vi "Tic-Tac-Toe-PerfectAI.vi"() -> ()   [LabVIEW 2013]
uses:
  Typedef/Board.ctl
  Typedef/Cell.ctl
  Typedef/AI Table Node.ctl
panel:
  in  "Blue AI":bool
  in  "Red AI":bool
  out "Blue":bool
  out "Red":bool
  out "Board":T1={"0,0"=enum."X", "1,0"=enum."X", "2,0"=enum."X", "0,1"=enum."X", "1,1"=enum."X", "2,1"=enum."X", "0,2"=enum."X", "1,2"=enum."", "2,2"=enum."X"}
  # "Turn"
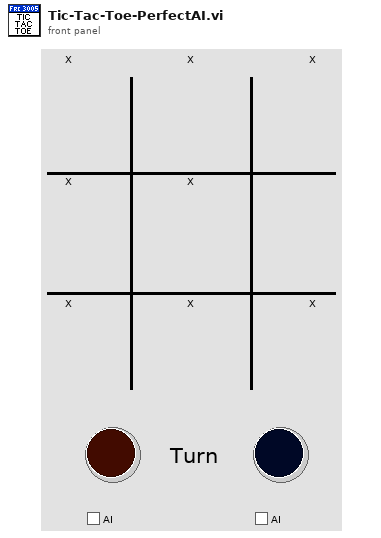
[diagram p1: front panel]
types:
  T1 = typedef "Board.ctl" = cluster{"0,0":T2, "1,0":T2, "2,0":T2, "0,1":T2, "1,1":T2, "2,1":T2, "0,2":T2, "1,2":T2, "2,2":T2}
  T2 = typedef "Cell.ctl" = enum16{"", "X", "O"}
  T3 = cluster{"Selected Row":i32, "Selected Column":i32, "Team":bool, "AI Table Head":i32, "AI Table Const":i32}
  T4 = typedef "AI Table Node.ctl" = cluster{"Board State":i32, "Child Nodes":i32[], "X PCT":dbl, "O PCT":dbl, "Index":i32}
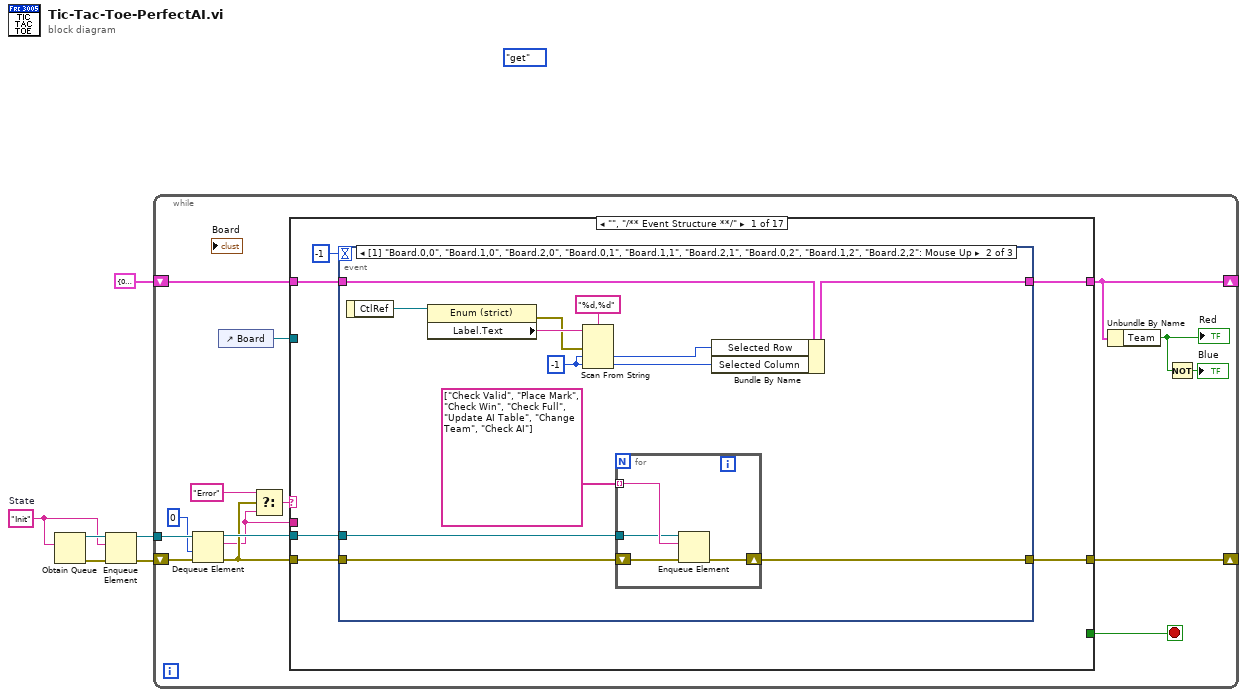
[diagram p0: block diagram]
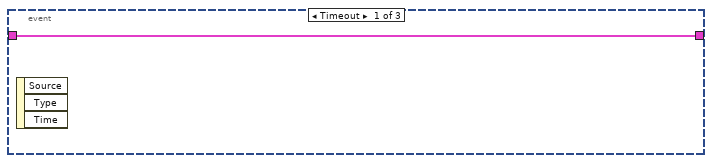
[diagram p2: hidden frame]
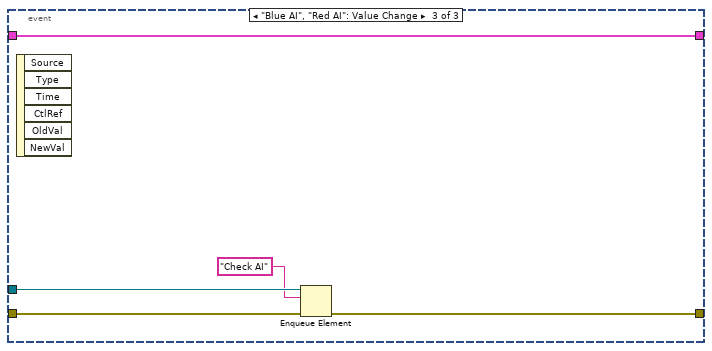
[diagram p3: hidden frame]
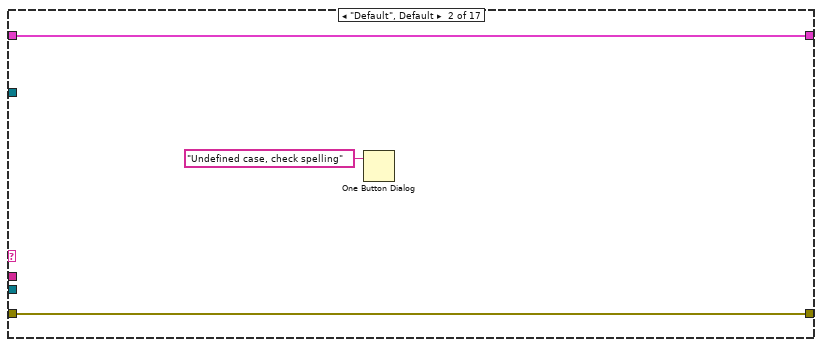
[diagram p4: hidden frame]
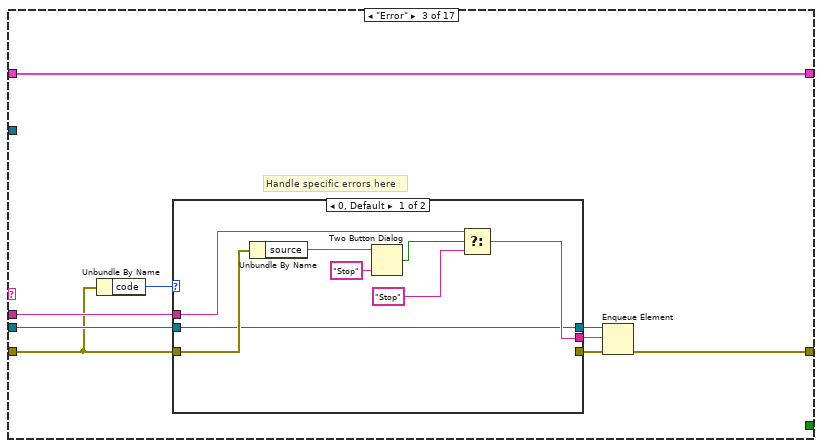
[diagram p5: hidden frame]
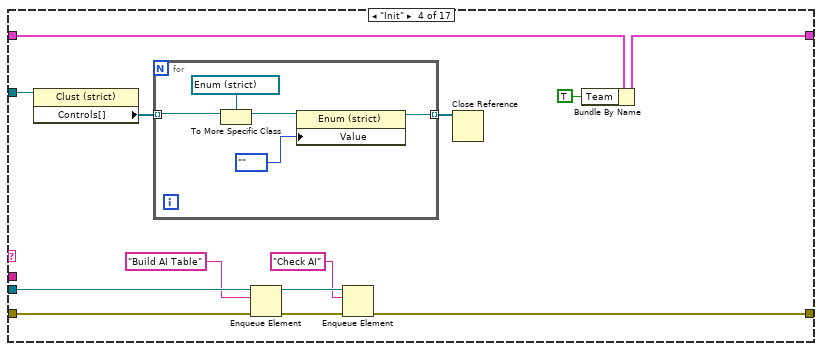
[diagram p7: hidden frame]
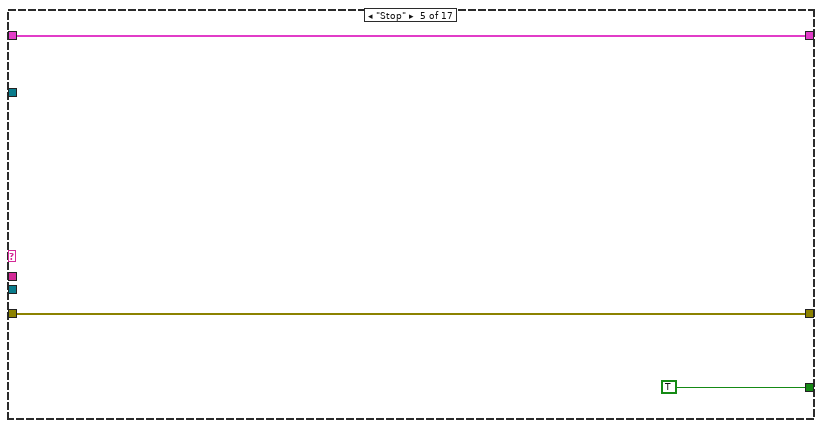
[diagram p8: hidden frame]
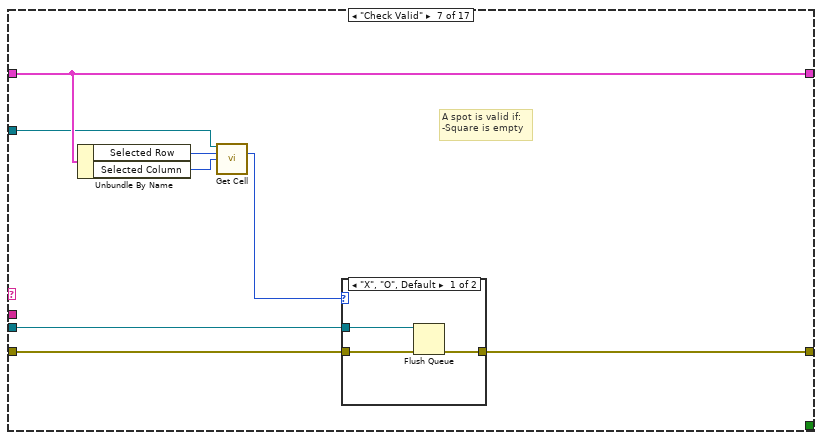
[diagram p10: hidden frame]
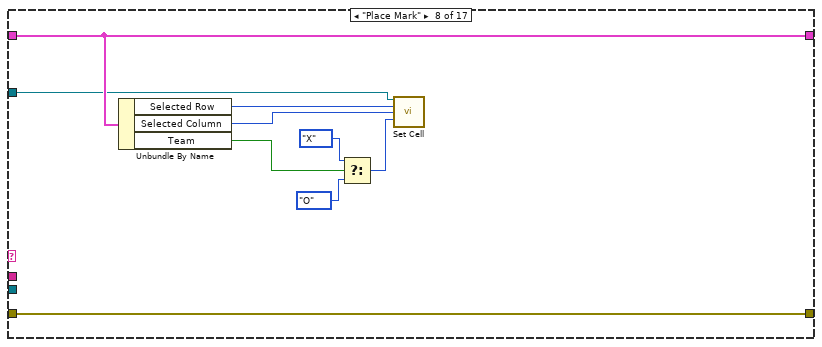
[diagram p12: hidden frame]
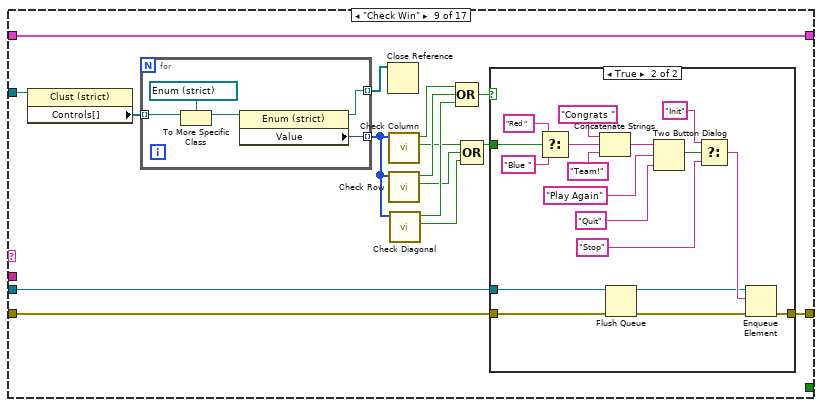
[diagram p13: hidden frame]
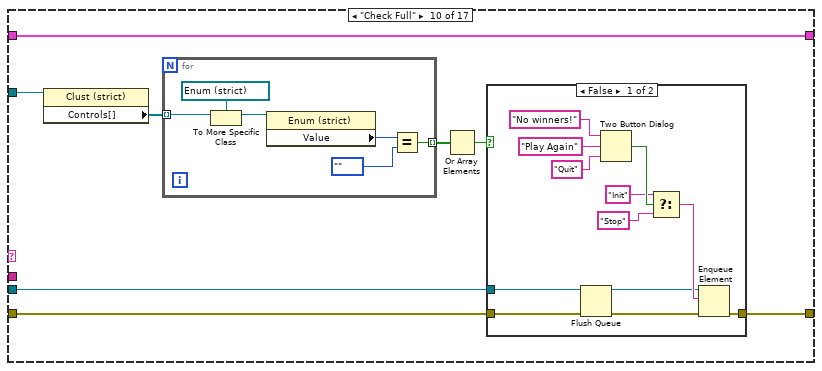
[diagram p15: hidden frame]
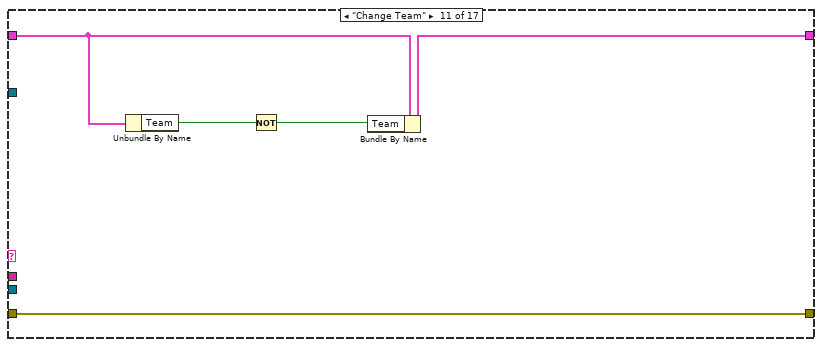
[diagram p17: hidden frame]
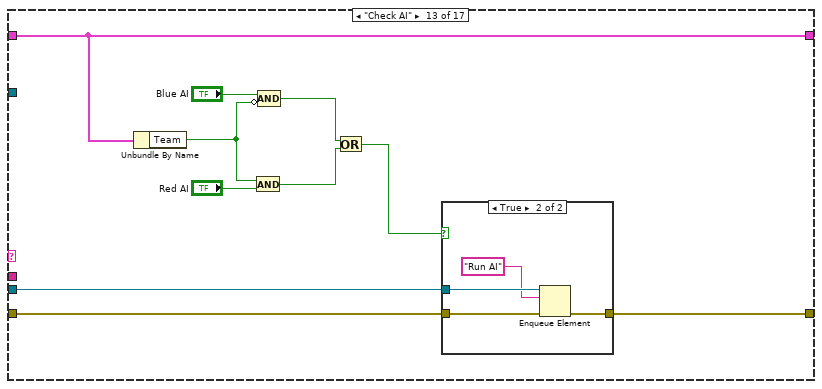
[diagram p19: hidden frame]
diagram:
  (unwired) enum16{"get", "set", "reset"}."get"
  w1 = "Init"  # State
  n1 = Obtain Queue(element data type=w1) -> (queue out=w2:refnum<queue>, error out=w3:errorcluster)  [unwired: 4 in, 1 out]
  n2 = Enqueue Element(queue=w2, element=w1, error in (no error)=w3) -> (queue out=w5:refnum<queue>, error out=w4:errorcluster)  [unwired: 1 in, 1 out]
  n3 = while {
    tunnel: w5 -> [w20]
    shift-right: [w19] -> _
    shift-left: w4 -> [w18]
    shift-right: [w9] -> _
    shift-left: T3 {"Selected Row"=0, "Selected Column"=0, "Team"=TRUE, "AI Table Head"=0, "AI Table Const"=0} -> [w13]
    stop <- w10 stop-if-true
    n4 = Dequeue Element(queue=w20, timeout in ms (-1)=0, error in (no error)=w18) -> (queue out=w21:refnum<queue>, element=w12:string, error out=w16:errorcluster)  [unwired: 1 out]
    n5 = control-ref of="Board"() -> (w11:refnum<vi>)
    n6 = Select(t="Error", s=w16, f=w12) -> (s? t:f=w17:string)
    n7 = case shown="\"\", \"/** Event Structure **/\"" w17 {
      tunnel: w21 -> [w22 _ w56 w79 _ _ w103 _ w127 w159 _ _ w193 w208 _ _ _]
      tunnel: w16 -> [w27 w52 w55 w80 w94 w96 w104 w117 w129 w160 w189 w191 w195 w211 w221 w233 w265]
      tunnel: [w26 w52 w61 w76 w94 w96 w102 w117 w128 w158 w189 w191 w194 w209 w221 w232 w265] -> w19
      tunnel: w13 -> [w24 w53 w62 w86 w93 w95 w101 w116 w133 w165 w187 w190 w201 w210 w219 w229 w264]
      tunnel: [w23 w53 w62 w83 w93 w95 w101 w116 w133 w165 w188 w190 w201 w210 w220 w228 w261] -> w9
      tunnel: w12 -> [_ _ w60 _ _ _ _ _ _ _ _ _ _ _ _ _ _]
      tunnel: w11 -> [_ _ _ w85 _ _ w98 w113 w132 w164 _ _ _ _ _ _ _]
      tunnel: [_ _ _ _ TRUE _ _ _ _ _ _ _ _ _ _ _ _] -> w10
      frame "", "/** Event Structure **/" {
        n8 = event shown="[1] \"Board.0,0\", \"Board.1,0\", \"Board.2,0\", \"Board.0,1\", \"Board.1,1\", \"Board.2,1\", \"Board.0,2\", \"Board.1,2\", \"Board.2,2\": Mouse Up" {
          selector: _ -> [_ _ _]
          dyn-events: _ -> [_ _ _]
          timeout: -1 -> [_ _ _]
          tunnel: w27 -> [_ w31 w49]
          tunnel: [_ w30 w47] -> w26
          tunnel: w24 -> [w28 w36 w46]
          tunnel: [w28 w35 w46] -> w23
          tunnel: w22 -> [_ w29 w50]
          event Timeout {
            n9 = event-data() -> ()  [unwired: 1 in, 3 out]
          }
          event Mouse Up {
            w37 = -1 ("default value 1")
            n10 = event-data() -> ("CtlRef"=w41:refnum<vi>)  [unwired: 1 in]
            n11 = property class="Enum (strict)"(reference=w41) -> (error out=w38:errorcluster, "Label.Text"=w40:string)  [unwired: 1 in, 1 out]
            n12 = Scan From String(format string="%d,%d", input string=w40, error in=w38, default 1=w37, default 2=w37) -> (output 1=w33:i32, output 2=w34:i32)  [unwired: 1 in, 3 out]
            n13 = for {
              tunnel: string[] ["Check Valid", "Place Mark", "Check Win", "Check Full", "Update AI Table", "Change Team", "Check AI"] -> [w45] mode=indexing
              shift-right: [w43] -> w30
              shift-left: w31 -> [w44]
              tunnel: w29 -> [w42]
              n14 = Enqueue Element(queue=w42, element=w45, error in (no error)=w44) -> (error out=w43:errorcluster)  [unwired: 1 in, 2 out]
            }
            n15 = Bundle By Name(cluster=w36, "Selected Row"=w33, "Selected Column"=w34) -> (w35:T3)
          }
          event "Blue AI", "Red AI": Value Change {
            n16 = event-data() -> ()  [unwired: 1 in, 6 out]
            n17 = Enqueue Element(queue=w50, element="Check AI", error in (no error)=w49) -> (error out=w47:errorcluster)  [unwired: 1 in, 2 out]
          }
        }
      }
      frame "Default", Default {
        n18 = One Button Dialog(message="Undefined case, check spelling") -> ()  [unwired: 1 in, 1 out]
      }
      frame "Error" {
        # "Handle specific errors here"
        n19 = Unbundle By Name(w55) -> ("code"=w54:i32)
        n20 = case shown="0, Default" w54 {
          tunnel: w60 -> [w70 w71]
          tunnel: [w69 w71] -> w59
          tunnel: w55 -> [w64 w72]
          tunnel: [_ w72] -> w58
          tunnel: [w63 w73] -> w57
          tunnel: w56 -> [w63 w73]
          frame 0, Default {
            n21 = Unbundle By Name(w64) -> ("source"=w66:string)
            n22 = Two Button Dialog(message=w66, 1:"Stop" ("F button name (\"Cancel\")")) -> (T button?=w68:bool)  [unwired: 1 in]
            n23 = Select(t=w70, s=w68, f="Stop") -> (s? t:f=w69:string)
          }
          frame 1 {
          }
        }
        n24 = Enqueue Element(queue=w57, element=w59, error in (no error)=w58) -> (error out=w61:errorcluster)  [unwired: 1 in, 2 out]
      }
      frame "Init" {
        n25 = property class="Clust (strict)"(reference=w85) -> ("Controls[]"=w84:refnum<vi>[])  [unwired: 1 in, 2 out]
        n26 = for {
          tunnel: w84 -> [w91] mode=indexing
          tunnel: [w87] -> w81 mode=indexing
          n27 = To More Specific Class(target class=refnum<vi> refnum ("1,2"), reference=w91) -> (specific class reference=w90:refnum<vi>)  [unwired: 1 in, 1 out]
          n28 = property class="Enum (strict)"(reference=w90, "Value"=Cell."") -> (reference out=w87:refnum<vi>)  [unwired: 1 in, 1 out]
        }
        n29 = Enqueue Element(queue=w79, element="Build AI Table", error in (no error)=w80) -> (queue out=w75:refnum<queue>, error out=w77:errorcluster)  [unwired: 1 in, 1 out]
        n30 = Enqueue Element(queue=w75, element="Check AI", error in (no error)=w77) -> (error out=w76:errorcluster)  [unwired: 1 in, 2 out]
        n31 = Close Reference(reference=w81) -> ()  [unwired: 1 in, 1 out]
        n32 = Bundle By Name(cluster=w86, "Team"=TRUE) -> (w83:T3)
      }
      frame "Stop" {
      }
      frame "/*** Game Functions ***/" {
      }
      frame "Check Valid" {
        # "A spot is valid if:\n-Square is empty"
        n33 = Unbundle By Name(w101) -> ("Selected Row"=w100:i32, "Selected Column"=w99:i32)
        n34 = call "Get Cell.vi"("Board ref in"=w98, "Row"=w100, "Column"=w99) -> ("Value"=w97:T2)  [unwired: 10 in, 2 out]
        n35 = case shown="\"X\", \"O\", Default" w97 {
          tunnel: w104 -> [w106 w108]
          tunnel: w103 -> [w107 _]
          tunnel: [w105 w108] -> w102
          frame "X", "O", Default {
            n36 = Flush Queue(queue=w107, error in (no error)=w106) -> (error out=w105:errorcluster)  [unwired: 2 out]
          }
          frame "" {
          }
        }
      }
      frame "Place Mark" {
        n37 = Unbundle By Name(w116) -> ("Selected Row"=w115:i32, "Selected Column"=w114:i32, "Team"=w109:bool)
        n38 = Select(t=Cell."X" ("Value"), s=w109, f=Cell."O" ("Value")) -> (s? t:f=w110:T2)
        n39 = call "Set Cell.vi"("Board ref in"=w113, "Row"=w115, "Column"=w114, "Value"=w110) -> ()  [unwired: 10 in, 2 out]
      }
      frame "Check Win" {
        n40 = property class="Clust (strict)"(reference=w132) -> ("Controls[]"=w131:refnum<vi>[])  [unwired: 1 in, 2 out]
        n41 = for {
          tunnel: w131 -> [w157] mode=indexing
          tunnel: [w154] -> w118 mode=indexing
          tunnel: [w153] -> w130 mode=indexing
          n42 = To More Specific Class(target class=refnum<vi> refnum ("1,2"), reference=w157) -> (specific class reference=w156:refnum<vi>)  [unwired: 1 in, 1 out]
          n43 = property class="Enum (strict)"(reference=w156) -> (reference out=w153:refnum<vi>, "Value"=w154:T2)  [unwired: 1 in, 1 out]
        }
        n44 = Close Reference(reference=w130) -> ()  [unwired: 1 in, 1 out]
        n45 = call "Check Column.vi"("Array"=w118) -> ("Team"=w121:bool, "Win?"=w126:bool)  [unwired: 9 in]
        n46 = call "Check Row.vi"("Array"=w118) -> ("Team"=w120:bool, "Win?"=w125:bool)  [unwired: 9 in]
        n47 = call "Check Diagonal.vi"("Array"=w118) -> ("Team"=w119:bool, "Win?"=w124:bool)  [unwired: 9 in]
        n48 = Compound Arithmetic op=OR(w126, w125, w124) -> (w123:bool)
        n49 = Compound Arithmetic op=OR(w121, w120, w119) -> (w122:bool)
        n50 = case shown="True" w123 {
          tunnel: w129 -> [w134 w152]
          tunnel: [w134 w142] -> w128
          tunnel: w122 -> [_ w145]
          tunnel: w127 -> [_ w136]
          frame False {
          }
          frame True {
            n51 = Select(t="Red " ("message"), s=w145, f="Blue " ("message")) -> (s? t:f=w146:string)
            n52 = Concatenate Strings("Congrats " ("message"), w146, "Team!" ("message")) -> (w149:string)
            n53 = Flush Queue(queue=w136, error in (no error)=w152) -> (queue out=w135:refnum<queue>, error out=w137:errorcluster)  [unwired: 1 out]
            n54 = Two Button Dialog(message=w149, 1:"Quit" ("message"), 2:"Play Again" ("message")) -> (T button?=w141:bool)
            n55 = Select(t="Init" ("message"), s=w141, f="Stop" ("message")) -> (s? t:f=w140:string)
            n56 = Enqueue Element(queue=w135, element=w140, error in (no error)=w137) -> (error out=w142:errorcluster)  [unwired: 1 in, 2 out]
          }
        }
      }
      frame "Check Full" {
        n57 = property class="Clust (strict)"(reference=w164) -> ("Controls[]"=w163:refnum<vi>[])  [unwired: 1 in, 2 out]
        n58 = for {
          tunnel: w163 -> [w183] mode=indexing
          tunnel: [w179] -> w162 mode=indexing
          n59 = To More Specific Class(target class=refnum<vi> refnum ("1,2"), reference=w183) -> (specific class reference=w182:refnum<vi>)  [unwired: 1 in, 1 out]
          n60 = property class="Enum (strict)"(reference=w182) -> ("Value"=w181:T2)  [unwired: 1 in, 2 out]
          n61 = Equal?(x=w181, y=Cell."") -> (x = y?=w179:bool)
        }
        n62 = Or Array Elements(Boolean array=w162) -> (logical OR=w161:bool)
        n63 = case shown="False" w161 {
          tunnel: w160 -> [w174 w178]
          tunnel: w159 -> [w167 _]
          tunnel: [w169 w178] -> w158
          frame False {
            n64 = Flush Queue(queue=w167, error in (no error)=w174) -> (queue out=w166:refnum<queue>, error out=w168:errorcluster)  [unwired: 1 out]
            n65 = Two Button Dialog(message="No winners!", 1:"Quit" ("T button name (\"OK\")"), 2:"Play Again" ("T button name (\"OK\")")) -> (T button?=w173:bool)
            n66 = Select(t="Init" ("T button name (\"OK\")"), s=w173, f="Stop" ("T button name (\"OK\")")) -> (s? t:f=w171:string)
            n67 = Enqueue Element(queue=w166, element=w171, error in (no error)=w168) -> (error out=w169:errorcluster)  [unwired: 1 in, 2 out]
          }
          frame True {
          }
        }
      }
      frame "Change Team" {
        n68 = Unbundle By Name(w187) -> ("Team"=w185:bool)
        n69 = Not(x=w185) -> (.not. x?=w186:bool)
        n70 = Bundle By Name(cluster=w187, "Team"=w186) -> (w188:T3)
      }
      frame "/*** AI Section ***/" {
      }
      frame "Check AI" {
        n71 = Unbundle By Name(w201) -> ("Team"=w198:bool)
        n72 = And(x=w198, y="Red AI") -> (x .and. y?=w196:bool)
        n73 = Compound Arithmetic op=AND("Blue AI", invert w198) -> (w199:bool)
        n74 = Or(x=w199, y=w196) -> (x .or. y?=w192:bool)
        n75 = case shown="True" w192 {
          tunnel: w195 -> [w202 w206]
          tunnel: [w202 w205] -> w194
          tunnel: w193 -> [_ w204]
          frame False {
          }
          frame True {
            n76 = Enqueue Element(queue=w204, element="Run AI", error in (no error)=w206) -> (error out=w205:errorcluster)  [unwired: 1 in, 2 out]
          }
        }
      }
      frame "Run AI" {
        n77 = for {
          shift-right: [w214] -> w209
          shift-left: w211 -> [w215]
          tunnel: w208 -> [w213]
          tunnel: string[] ["Pick Move", "Place Mark", "Check Win", "Check Full", "Change Team", "Check AI"] -> [w212] mode=indexing
          n78 = Enqueue Element(queue=w213, element=w212, error in (no error)=w215) -> (error out=w214:errorcluster)  [unwired: 1 in, 2 out]
        }
      }
      frame "Build AI Table" {
        n79 = Unbundle By Name(w219) -> ("AI Table Const"=w217:i32)
        n80 = Equal To 0?(x=w217) -> (x = 0?=w218:bool)
        n81 = case shown="True" w218 {
          tunnel: w217 -> [w222 _]
          tunnel: [w222 w223] -> w216
          frame False {
          }
          frame True {
            n82 = New Data Value Reference(data value=T4 {"Board State"=0, "Child Nodes"=[], "X PCT"=0.0, "O PCT"=0.0, "Index"=0}) -> (data value reference=w226:refnum<data-value>)  [unwired: 1 in, 1 out]
            n83 = Type Cast(type=0, x=w226) -> (*(type *) &x=w225:i32)
            n84 = call "Build AI Table.vi"("AI Node Ref In"=w225) -> ("AI Node Ref Out"=w223:i32)  [unwired: 8 in, 2 out]
          }
        }
        n85 = Bundle By Name(cluster=w219, "AI Table Const"=w216, "AI Table Head"=w216) -> (w220:T3)
      }
      frame "Update AI Table" {
        w240 = refnum<data-value> refnum ("data value reference")
        # "Update the AI table after a human move"
        n86 = Unbundle By Name(w229) -> ("AI Table Head"=w242:i32, "Selected Column"=w236:i32, "Selected Row"=w238:i32)
        n87 = Multiply(x=w238, y=3) -> (x*y=w237:i32)
        n88 = Type Cast(type=w240, x=w242) -> (*(type *) &x=w241:refnum<data-value>)
        n89 = Add(x=w236, y=w237) -> (x+y=w235:i32)
        n90 = in-place {
          in-place-border: w240 -> [w247]
          in-place-border: w235 -> [w245]
          in-place-border: [w244] -> w234
          in-place-border: [w243] -> w230
          n91 = in-place-dvr #1(w241) -> (w246:T4)  [unwired: 1 out]
          n92 = Unbundle By Name(w246) -> ("Child Nodes"=w248:i32[])
          n93 = for {
            tunnel: w248 -> [w249] mode=indexing
            tunnel: w247 -> [w253]
            tunnel: w245 -> [w251]
            tunnel: [w250] -> w244
            tunnel: [w249] -> w243
            stop <- w250 stop-if-true
            n94 = Type Cast(type=w253, x=w249) -> (*(type *) &x=w252:refnum<data-value>)
            n95 = in-place {
              in-place-border: w251 -> [w256]
              in-place-border: [w255] -> w250
              n96 = in-place-dvr #2(w252) -> (w254:T4)  [unwired: 1 out]
              n97 = Unbundle By Name(w254) -> ("Index"=w257:i32)
              n98 = Equal?(x=w257, y=w256) -> (x = y?=w255:bool)
              n99 = in-place-dvr #2(w254) -> ()  [unwired: 2 out]
            }
          }
          n100 = in-place-dvr #1(w246) -> ()  [unwired: 2 out]
        }
        n101 = Bundle By Name(cluster=w229, "AI Table Head"=w230) -> (w228:T3)
        n102 = Select(t=w233, s=w234, f=errorcluster {"status"=TRUE, "code"=5001, "source"="Something went wrong"} ("error out")) -> (s? t:f=w232:errorcluster)
      }
      frame "Pick Move" {
        n103 = Unbundle By Name(w264) -> ("AI Table Head"=w263:i32, "Team"=w262:bool)
        n104 = call "Pick AI Move.vi"("Team"=w262, "AI Table Head"=w263) -> ("Selected Col"=w258:i32, "Selected Row"=w259:i32, "AI Table Child"=w260:i32)  [unwired: 6 in, 1 out]
        n105 = Bundle By Name(cluster=w264, "AI Table Head"=w260, "Selected Row"=w259, "Selected Column"=w258) -> (w261:T3)
      }
    }
    n106 = Unbundle By Name(w9) -> ("Team"=w8:bool)
    "Red" <- w8
    n107 = Not(x=w8) -> (.not. x?=→"Blue":bool)
  }
